vi "Field Draw Target.vi"(4 "Lado":enum16{"Esquerdo", "Direito"}(ring) caption="Enum", 6 "Draw Targets?":T1, 8 "picture in":picture, 9 "Offset":T6, 10 "Scale mm/pixel":dbl, 11 "Robot":T3={"id"=0, "function"=enum."Attacker", "x"=0.0, "y"=0.0, "orientation"=0.0, "v_tangent"=0.0, "v_normal"=0.0, "v_ang"=0.0, "kick_x"=0.0, "kick_z"=0.0, "dribble"=FALSE, "Timestamp"=timestamp(0 s since 1904-01-01), "dest_x"=0.0, "dest_y"=0.0, "dest_orientation"=0.0, "estimatives"={"est_v_tangent"=0.0, "est_v_normal"=0.0, "est_vx"=0.0, "est_vy"=0.0, "Pos Robot Est"=[]}, "dest_x_kick"=0.0, "dest_y_kick"=0.0, "Gap Coord"=[], "States"=enum."GoToTangent"}) -> (0 "picture out":picture)   [LabVIEW 2017]
uses:
  <vilib>/Utility/miscctls.llb/LVBoundsTypeDef.ctl
  Core/AI Robot.ctl
  Intel/Functions Enum.ctl
  Intel/AttackerStates.ctl
  <vilib>/Analysis/coordinate.llb/Angle Range (Degree).ctl
  DrawTargets.ctl
  <vilib>/Analysis/coordinate.llb/2D Cartesian Coordinate Rotation (Scalar).vi
  <vilib>/Analysis/NI_AAL_Angle.lvlib
  <vilib>/Analysis/coordinate.llb/Wrap Angle (scalar).vi
  <vilib>/Analysis/NI_AALPro.lvlib
panel:
  in  "angle range":T2=1
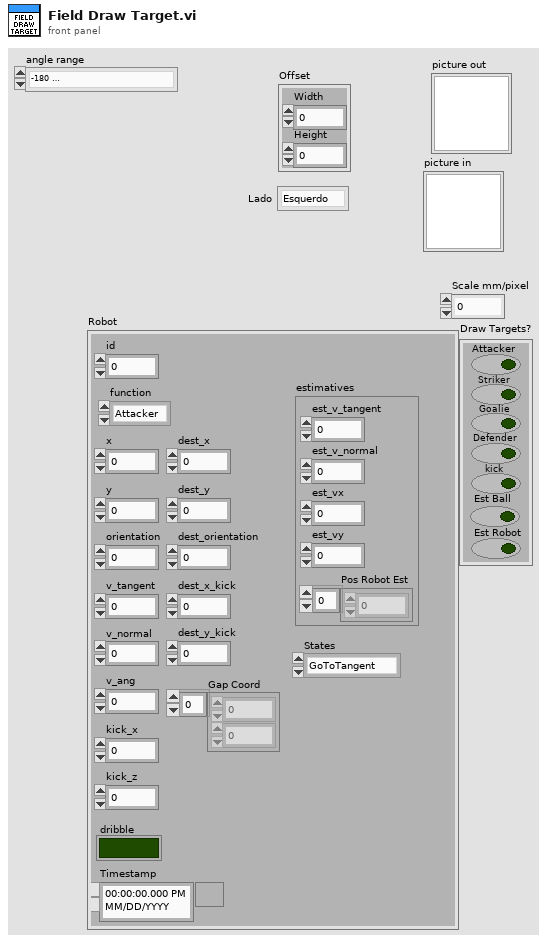
[diagram p1: front panel]
types:
  T1 = typedef "DrawTargets.ctl" = cluster{"Attacker":bool, "Striker":bool, "Goalie":bool, "Defender":bool, "kick":bool, "Est Ball":bool, "Est Robot":bool}
  T2 = typedef "NI_AAL_Angle.lvlib/Angle Range (Degree).ctl" = u16
  T3 = typedef "AI Robot.ctl" = cluster{"id":u32, "function":T4, "x":dbl, "y":dbl, "orientation":dbl, "v_tangent":dbl, "v_normal":dbl, "v_ang":dbl, "kick_x":dbl, "kick_z":dbl, "dribble":bool, "Timestamp":timestamp, "dest_x":dbl, "dest_y":dbl, "dest_orientation":dbl, "estimatives":cluster{"est_v_tangent":dbl, "est_v_normal":dbl, "est_vx":dbl, "est_vy":dbl, "Pos Robot Est":dbl[]}, "dest_x_kick":dbl, "dest_y_kick":dbl, "Gap Coord":dbl[], "States":T5}
  T4 = typedef "Functions Enum.ctl" = enum16{"Attacker", "Goalie", "Defender", "Striker", "Goto 0", "Dummy", "Kicker", "ZigZag"}
  T5 = typedef "AttackerStates.ctl" = enum16{"Pass", "GoToTangent", "BallGetting", "GoToKick", ""}
  T6 = typedef "LVBoundsTypeDef.ctl" = cluster{"Width":u32, "Height":u32}
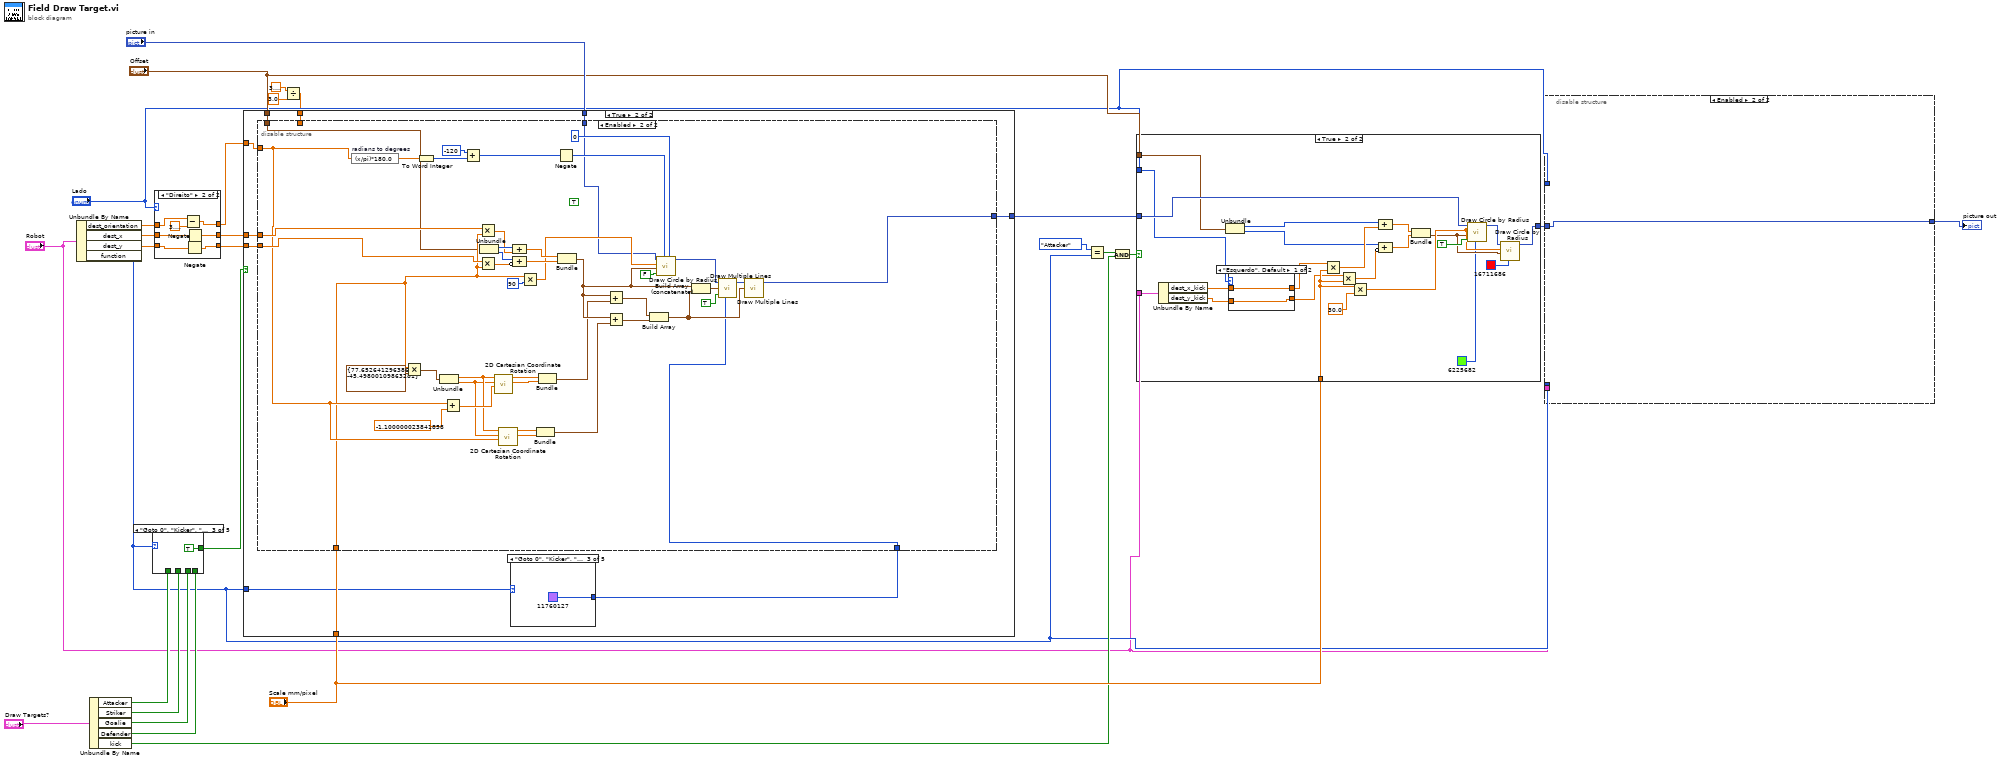
[diagram p0: block diagram]
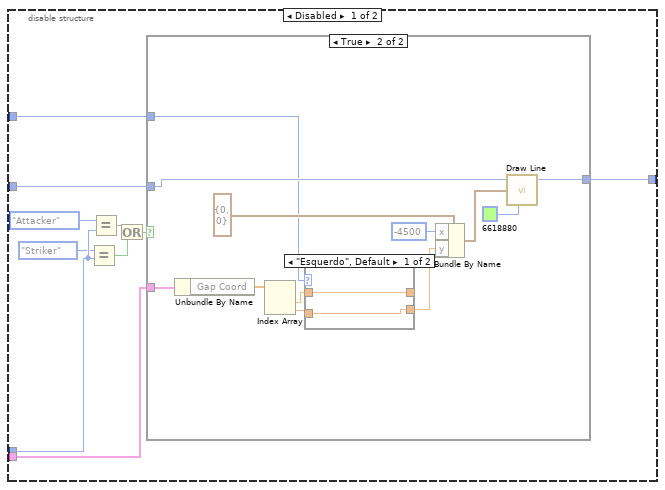
[diagram p2: hidden frame]
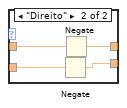
[diagram p4: hidden frame]
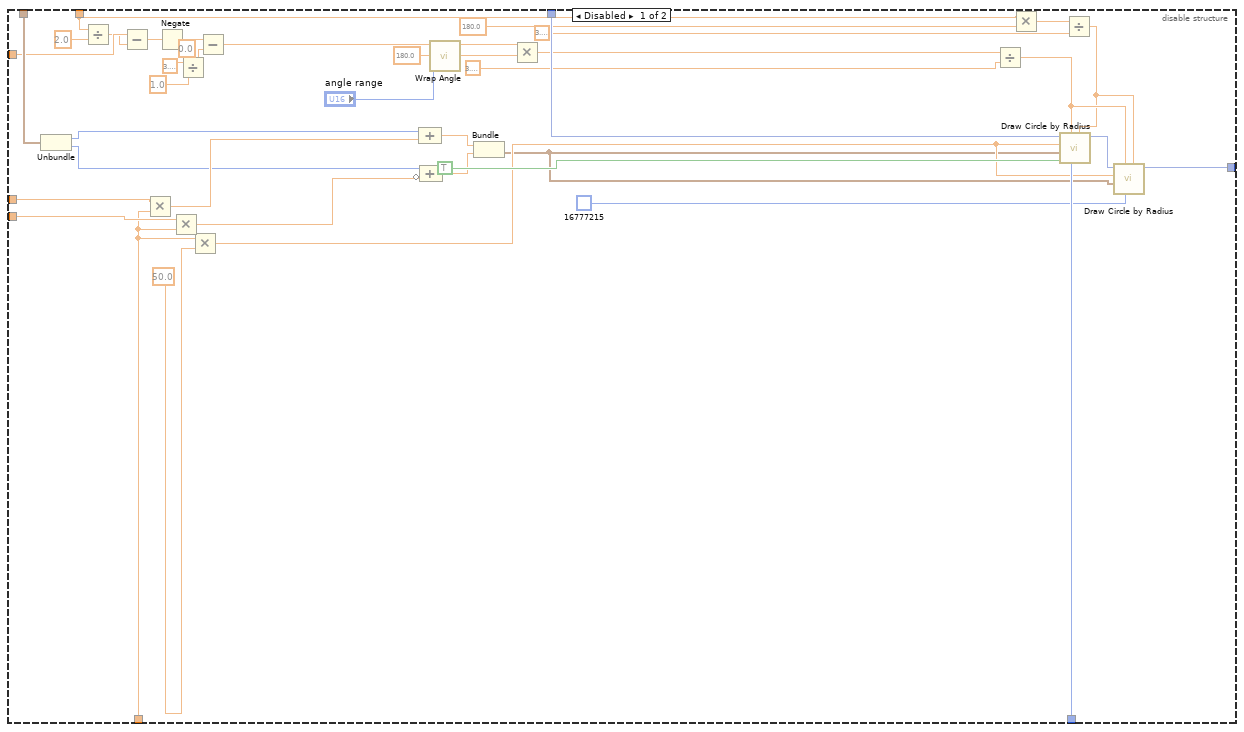
[diagram p11: hidden frame]
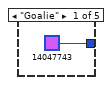
[diagram p12: hidden frame]
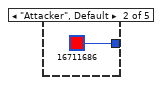
[diagram p13: hidden frame]
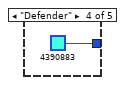
[diagram p14: hidden frame]
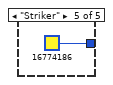
[diagram p15: hidden frame]
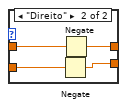
[diagram p17: hidden frame]
diagram:
  n1 = Unbundle By Name("Robot") -> ("dest_orientation"=w6:dbl, "dest_x"=w14:dbl, "dest_y"=w13:dbl, "function"=w10:T4)
  n2 = Unbundle By Name("Draw Targets?") -> ("Attacker"=w21:bool, "Striker"=w22:bool, "Goalie"=w20:bool, "Defender"=w23:bool, "kick"=w18:bool)
  n3 = case shown="\"Goto 0\", \"Kicker\", \"ZigZag\"" w10 {
    tunnel: [w29 w30 TRUE ("Draw Target Striker?") w32 w33] -> w24
    tunnel: w23 -> [_ _ _ w32 _]
    tunnel: w22 -> [_ _ _ _ w33]
    tunnel: w21 -> [w29 _ _ _ _]
    tunnel: w20 -> [_ w30 _ _ _]
    frame "Attacker", Default {
    }
    frame "Goalie" {
    }
    frame "Goto 0", "Kicker", "ZigZag" {
    }
    frame "Defender" {
    }
    frame "Striker" {
    }
  }
  n4 = case shown="\"Direito\"" "Lado" {
    tunnel: [w36 w43] -> w15
    tunnel: w14 -> [w36 w40]
    tunnel: [w35 w41] -> w12
    tunnel: w13 -> [w35 w42]
    tunnel: w6 -> [w34 w38]
    tunnel: [w34 w39] -> w5
    frame "Esquerdo", Default {
    }
    frame "Direito" {
      n5 = Subtract(x=w38, y=3.141592653589793) -> (x-y=w39:dbl)
      n6 = Negate(x=w42) -> (-x=w41:dbl)
      n7 = Negate(x=w40) -> (-x=w43:dbl)
    }
  }
  n8 = Divide(x=3.141592653589793, y=3.0) -> (x/y=w4:dbl)
  n9 = case shown="True" w24 {
    tunnel: w12 -> [_ w53]
    tunnel: w15 -> [_ w52]
    tunnel: "picture in" -> [w44 w51]
    tunnel: [w44 w50] -> w27
    tunnel: "Offset" -> [_ w49]
    tunnel: "Scale mm/pixel" -> [_ w48]
    tunnel: w10 -> [_ w47]
    tunnel: w5 -> [_ w46]
    tunnel: w4 -> [_ w45]
    frame False {
    }
    frame True {
      n10 = case shown="\"Goto 0\", \"Kicker\", \"ZigZag\"" w47 {
        tunnel: [u32 14047743 ("color(black)") u32 16711686 ("color(black)") u32 11760127 ("color(black)") u32 4390883 ("color(black)") u32 16774186 ("color(black)")] -> w54
        frame "Goalie" {
        }
        frame "Attacker", Default {
        }
        frame "Goto 0", "Kicker", "ZigZag" {
        }
        frame "Defender" {
        }
        frame "Striker" {
        }
      }
      n11 = disable-structure shown="Enabled" {
        disable-tunnel: w54 -> [w92 w95]
        disable-tunnel: w53 -> [w90 w100]
        disable-tunnel: w52 -> [w89 w101]
        disable-tunnel: w51 -> [w82 w98]
        disable-tunnel: [w78 w97] -> w50
        disable-tunnel: w49 -> [w77 w94]
        disable-tunnel: w48 -> [w76 w96]
        disable-tunnel: w46 -> [w67 w99]
        disable-tunnel: w45 -> [w64 _]
        frame Disabled {
          (unwired) 0.0 ("y")
          n12 = Unbundle(w77) -> ("Width"=w88:u32, "Height"=w85:u32)
          n13 = Divide(x=w64, y=2.0) -> (x/y=w66:dbl)
          n14 = Subtract(x=w67, y=w66) -> (x-y=w73:dbl)
          n15 = Multiply(x=w89, y=w76) -> (x*y=w87:dbl)
          n16 = Negate(x=w73) -> (-x=w72:dbl)
          n17 = Multiply(x=w90, y=w76) -> (x*y=w84:dbl)
          n18 = Divide(x=3.141592653589793, y=1.0) -> (x/y=w55:dbl)
          n19 = Multiply(x=w76, y=sgl 50.0 ("radius")) -> (x*y=w80:dbl)
          n20 = Subtract(x=w72, y=w55) -> (x-y=w68:dbl)
          n21 = Compound Arithmetic op=ADD(w88, w87) -> (w86:dbl)
          n22 = Compound Arithmetic op=ADD(w85, invert w84) -> (w83:dbl)
          n23 = call-poly <vilib>:"Wrap Angle.vi"("angle range"="angle range", "angle in"=w68) -> ("angle out"=w65:dbl)  [unwired: 8 in, 1 out]
          n24 = Bundle(w86, w83) -> (w79:cluster{dbl, dbl})  [unwired: 1 in]
          n25 = Multiply(x=w65, y=180.0) -> (x*y=w62:dbl)
          n26 = Divide(x=w62, y=3.141592653589793) -> (x/y=w57:dbl)
          n27 = Multiply(x=w64, y=180.0) -> (x*y=w63:dbl)
          n28 = Divide(x=w63, y=3.141592653589793) -> (x/y=w56:dbl)
          n29 = call <vilib>:"Draw Circle by Radius.vi"("arc size(360)"=w56, "color(black)"=w92, "start angle(0)"=w57, "fill?(F)"=TRUE, "pixel center"=w79, "radius"=w80, "picture"=w82) -> ("new picture"=w81:picture)  [unwired: 4 in]
          n30 = call <vilib>:"Draw Circle by Radius.vi"("arc size(360)"=w56, "color(black)"=u32 16777215, "start angle(0)"=w57, "pixel center"=w79, "radius"=w80, "picture"=w81) -> ("new picture"=w78:picture)  [unwired: 5 in]
        }
        frame Enabled {
          (unwired) TRUE ("fill?(F)")
          n31 = expression code="(x/pi)*180.0" "radians to degrees"(w99) -> (w128:dbl)
          n32 = Multiply(x=w96, y=cluster{sgl, sgl} {77.65264, -45.498} ("appended array")) -> (x*y=w107:cluster{dbl, dbl})
          n33 = To Word Integer(number=w128) -> (16bit integer=w127:i16)
          n34 = Unbundle(w107) -> (w112:dbl, w111:dbl)
          n35 = Add(x=w99, y=sgl -1.1 ("theta")) -> (x+y=w113:dbl)
          n36 = Add(x=i16 -120, y=w127) -> (x+y=w126:i16)
          n37 = Multiply(x=w101, y=w96) -> (x*y=w134:dbl)
          n38 = Multiply(x=w100, y=w96) -> (x*y=w131:dbl)
          n39 = Unbundle(w94) -> ("Width"=w135:u32, "Height"=w132:u32)
          n40 = call-poly <vilib>:"2D Cartesian Coordinate Rotation.vi"("theta"=w113, "y"=w111, "x"=w112) -> ("y out"=w115:dbl, "x out"=w116:dbl)  [unwired: 6 in, 1 out]
          n41 = call-poly <vilib>:"2D Cartesian Coordinate Rotation.vi"("theta"=w99, "y"=w111, "x"=w112) -> ("y out"=w109:dbl, "x out"=w110:dbl)  [unwired: 6 in, 1 out]
          n42 = Compound Arithmetic op=ADD(w135, w134) -> (w133:dbl)
          n43 = Compound Arithmetic op=ADD(w132, invert w131) -> (w130:dbl)
          n44 = Multiply(x=w96, y=i16 90 ("radius")) -> (x*y=w122:dbl)
          n45 = Bundle("x out"=w110, "y out"=w109) -> (w106:cluster{"x out":dbl, "y out":dbl})  [unwired: 1 in]
          n46 = Bundle("x out"=w116, "y out"=w115) -> (w105:cluster{"x out":dbl, "y out":dbl})  [unwired: 1 in]
          n47 = Negate(x=w126) -> (-x=w124:i16)
          n48 = Bundle(w133, w130) -> (w121:cluster{dbl, dbl})  [unwired: 1 in]
          n49 = Add(x=w121, y=w105) -> (x+y=w103:cluster{dbl, dbl})
          n50 = Add(x=w121, y=w106) -> (x+y=w104:cluster{dbl, dbl})
          n51 = Build Array(w103, w104) -> (w120:cluster{dbl, dbl}[])
          n52 = call <vilib>:"Draw Circle by Radius.vi"("arc size(360)"=i16 0, "start angle(0)"=w124, "fill?(F)"=FALSE, "pixel center"=w121, "radius"=w122, "picture"=w98) -> ("new picture"=w102:picture)  [unwired: 5 in]
          n53 = Build Array (concatenate)(w121, w120) -> (w118:cluster{dbl, dbl}[])
          n54 = call <vilib>:"Draw Multiple Lines.vi"("picture"=w102, "line endpoints"=w118, "fill?(F)"=TRUE, "color(black)"=w95) -> ("new picture"=w119:picture)  [unwired: 5 in]
          n55 = call <vilib>:"Draw Multiple Lines.vi"("picture"=w119, "line endpoints"=w120) -> ("new picture"=w97:picture)  [unwired: 7 in]
        }
      }
    }
  }
  n56 = Equal?(x=Functions_Enum."Attacker" ("y"), y=w10) -> (x = y?=w17:bool)
  n57 = And(x=w17, y=w18) -> (x .and. y?=w19:bool)
  n58 = case shown="True" w19 {
    tunnel: w27 -> [w142 w154]
    tunnel: [w142 w153] -> w11
    tunnel: "Robot" -> [_ w152]
    tunnel: "Offset" -> [_ w151]
    tunnel: "Scale mm/pixel" -> [_ w150]
    tunnel: "Lado" -> [_ w143]
    frame False {
    }
    frame True {
      n59 = Unbundle By Name(w152) -> ("dest_x_kick"=w147:dbl, "dest_y_kick"=w144:dbl)
      n60 = Unbundle(w151) -> ("Width"=w163:u32, "Height"=w160:u32)
      n61 = case shown="\"Esquerdo\", Default" w143 {
        tunnel: [w167 w171] -> w146
        tunnel: w147 -> [w167 w169]
        tunnel: [w166 w170] -> w145
        tunnel: w144 -> [w166 w168]
        frame "Esquerdo", Default {
        }
        frame "Direito" {
          n62 = Negate(x=w168) -> (-x=w170:dbl)
          n63 = Negate(x=w169) -> (-x=w171:dbl)
        }
      }
      n64 = Multiply(x=w146, y=w150) -> (x*y=w162:dbl)
      n65 = Multiply(x=w145, y=w150) -> (x*y=w159:dbl)
      n66 = Multiply(x=w150, y=sgl 30.0 ("radius")) -> (x*y=w156:dbl)
      n67 = Compound Arithmetic op=ADD(w163, w162) -> (w161:dbl)
      n68 = Compound Arithmetic op=ADD(w160, invert w159) -> (w158:dbl)
      n69 = Bundle(w161, w158) -> (w155:cluster{dbl, dbl})  [unwired: 1 in]
      n70 = call <vilib>:"Draw Circle by Radius.vi"("color(black)"=u32 6225682, "fill?(F)"=TRUE, "pixel center"=w155, "radius"=w156, "picture"=w154) -> ("new picture"=w157:picture)  [unwired: 6 in]
      n71 = call <vilib>:"Draw Circle by Radius.vi"("color(black)"=u32 16711686, "pixel center"=w155, "radius"=w156, "picture"=w157) -> ("new picture"=w153:picture)  [unwired: 7 in]
    }
  }
  n72 = disable-structure shown="Enabled" {
    disable-tunnel: w11 -> [w181 w201]
    disable-tunnel: w10 -> [w180 _]
    disable-tunnel: [w174 w201] -> w9
    disable-tunnel: "Robot" -> [w173 _]
    disable-tunnel: "Lado" -> [w172 _]
    frame Disabled {
      n73 = Equal?(x=Functions_Enum."Striker", y=w180) -> (x = y?=w175:bool)
      n74 = Equal?(x=Functions_Enum."Attacker", y=w180) -> (x = y?=w176:bool)
      n75 = Or(x=w176, y=w175) -> (x .or. y?=w177:bool)
      n76 = case shown="True" w177 {
        tunnel: w181 -> [w182 w190]
        tunnel: [w182 w191] -> w174
        tunnel: w173 -> [_ w194]
        tunnel: w172 -> [_ w184]
        frame False {
        }
        frame True {
          n77 = Unbundle By Name(w194) -> ("Gap Coord"=w192:dbl[])
          n78 = Index Array(array=w192) -> (element #1=w187:dbl, element #2=w186:dbl)  [unwired: 2 in]
          n79 = case shown="\"Esquerdo\", Default" w184 {
            tunnel: [w196 w200] -> _
            tunnel: w187 -> [w196 w198]
            tunnel: [w195 w199] -> w185
            tunnel: w186 -> [w195 w197]
            frame "Esquerdo", Default {
            }
            frame "Direito" {
              n80 = Negate(x=w197) -> (-x=w199:dbl)
              n81 = Negate(x=w198) -> (-x=w200:dbl)
            }
          }
          n82 = Bundle By Name(cluster=cluster{"x":i16, "y":i16} {"x"=0, "y"=0} ("end point"), "x"=i16 -4500, "y"=w185) -> (w189:cluster{"x":i16, "y":i16})
          n83 = call <vilib>:"Draw Line.vi"("picture"=w190, "end point"=w189, "color(black)"=u32 6618880) -> ("new picture"=w191:picture)  [unwired: 6 in]
        }
      }
    }
    frame Enabled {
    }
  }
  "picture out" <- w9
